vi "TEMPLATE_Constructor.vi"(8 "Error In":errorcluster) -> (0 "Error Out":errorcluster, 3 "New %TYPE%":refnum<class "LQIdentity.lvclass">)   [LabVIEW 2014, in "Template.lvlib" / "LQIdentity.lvclass"]
uses:
  LQIdentity.lvclass
  LQCoreEngine/_Internal/LQIdentity Registry Action.ctl
  LQIdentity.lvclass/LQIdentity.ctl
  Template.lvlib
  LQCoreEngine/LQCoreEngine.lvclass
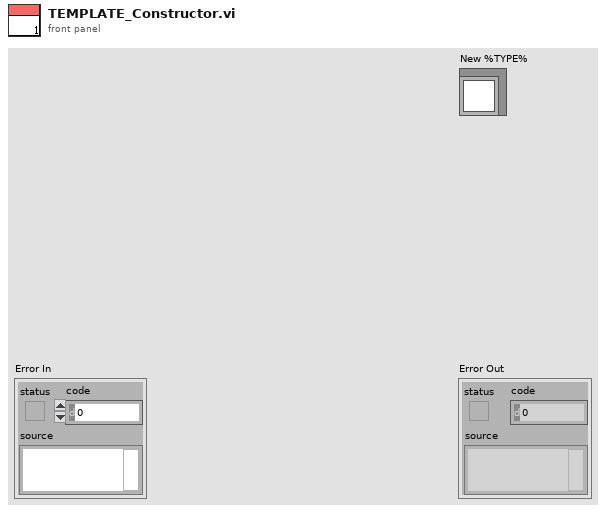
[diagram p1: front panel]
types:
  T1 = typedef "Template.lvlib/LQCoreEngine.lvclass/LQIdentity Registry Action.ctl" = enum16{"Init", "Register LQIdentity", "Get LQIdentity Info", "Deregister LQIdentity"}
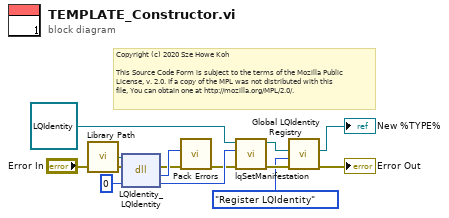
[diagram p0: block diagram]
diagram:
  # "Copyright (c) 2020 Sze Howe Koh\n\nThis Source Code Form is subject to the terms of the Mozilla Public\nLicense, v. 2.0. If a copy of the MPL was not distributed with this\nfile, You can obtain one at http://mozilla.org/MPL/2.0/."
  n1 = call "Library Path.vi"() -> ("Library Path"=w10:path)
  n2 = dll-call lib="?" fn="LQIdentity_LQIdentity"(path in=w10, error in="Error In", "_instance"=u64 0) -> (error out=w8:errorcluster, "errorCode"=w9:i32, "_instance"=w11:u64)  [unwired: 1 in, 1 out]
  n3 = call "Pack Errors.vi"("Error In"=w8, "Error Code"=w9) -> ("Error Out"=w7:errorcluster)  [unwired: 9 in]
  n4 = call "lqSetManifestation.vi"("Error In"=w7, "Manifestation"=w11, "LQIdentity in"=refnum<class "LQIdentity.lvclass"> refnum ("%TYPE%")) -> ("Error Out"=w5:errorcluster, "LQIdentity out"=w6:refnum<class "LQIdentity.lvclass">)  [unwired: 7 in]
  n5 = call "Global LQIdentity Registry.vi"("Error In"=w5, "Registry Action"=LQIdentity_Registry_Action."Register LQIdentity", "LQIdentity Info In"=w6) -> ("Error Out"=→"Error Out":errorcluster, "LQIdentity Info Out"=→"New %TYPE%":refnum<class "LQIdentity.lvclass">)  [unwired: 7 in]
